vi "ScreenSaverEnabled.vi"(8 "No Error":errorcluster) -> (0 "Error Out":errorcluster, 3 "Enabled?":bool)   [LabVIEW 2026, in "SDL3.lvlib" / "Video.lvlib"]
doc: "<B>Summary</B>\nCheck whether the screensaver is currently enabled.\n\n<B>Remarks</B>\nThe screensaver is disabled by default.\n\nThe default can also be changed using <B>SDL_HINT_VIDEO_ALLOW_SCREENSAVER</B>."
uses:
  Video.lvlib
  Lib/SDL3.dll
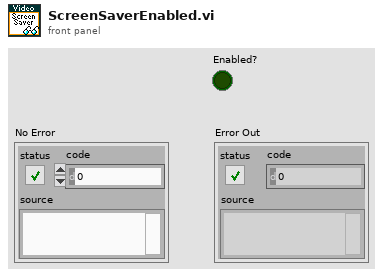
[diagram p1: front panel]
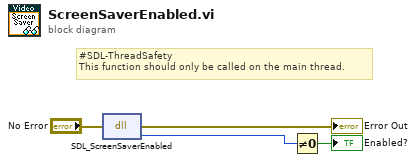
[diagram p0: block diagram]
diagram:
  # "#SDL-ThreadSafety\nThis function should only be called on the main thread."
  n1 = dll-call lib="C:/Users/saukko/Dev/LV-SDL3/Sources/SDL3/Lib/SDL3.*" fn="SDL_ScreenSaverEnabled"(error in="No Error") -> (error out=→"Error Out":errorcluster, "return type"=w1:i32)  [unwired: 2 in, 1 out]
  n2 = Not Equal To 0?(x=w1) -> (x != 0?=→"Enabled?":bool)
